vi "LED - Error Status.vi"(8 "Error In":errorcluster) -> (0 "Error Out":errorcluster)   [LabVIEW 2019]
uses:
  <vilib>/NI_Real-Time Target Support.lvlib
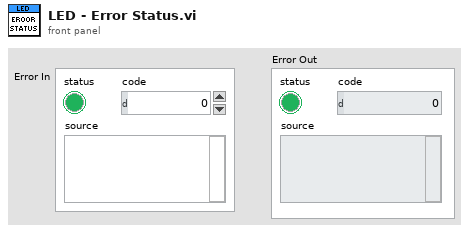
[diagram p1: front panel]
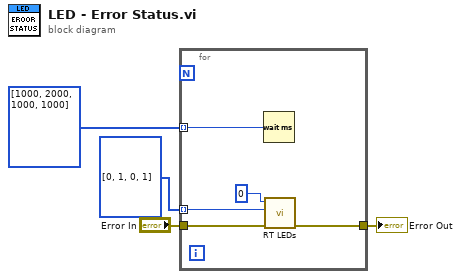
[diagram p0: block diagram]
diagram:
  n1 = for {
    tunnel: "Error In" -> [w8]
    tunnel: [w9] -> w3
    tunnel: u32[] [1000, 2000, 1000, 1000] ("milliseconds to wait") -> [w6] mode=indexing
    tunnel: i32[] [0, 1, 0, 1] ("State") -> [w5] mode=indexing
    n2 = Wait (ms)(milliseconds to wait=w6) -> ()  [unwired: 1 out]
    n3 = call <vilib>:"RT LEDs.vi"("error in (no error)"=w8, "State"=w5, "LED Num"=0) -> ("error out"=w9:errorcluster)  [unwired: 3 in, 1 out]
  }
  "Error Out" <- w3
